vi "Get Caster Wheel Click Zones.vi"(6 "wheel frame angle (rad)":dbl, 7 "global wheel position":cluster{"x":dbl, "y":dbl}, 8 "error in (no error)":errorcluster, 9 "wheel index":i32, 11 "wheel in":refnum<class "NI_Robotics_Wheel.lvclass">) -> (0 "error out":errorcluster, 2 "click zones":T1[](array[typedef]), 3 "wheel out":refnum<class "NI_Robotics_Wheel.lvclass">)   [LabVIEW 2017, in "NI_Robotics_Configure Steering Frame.lvlib"]
uses:
  <vilib>/robotics/Dialog/Configure Steering Frame/NI_Robotics_Configure Steering Frame.lvlib
  <vilib>/robotics/Dialog/Configure Steering Frame/Click Zone.ctl
  <vilib>/robotics/Steering/Wheel/NI_Robotics_Wheel.lvclass
  <vilib>/Analysis/coordinate.llb/2D Cartesian Coordinate Rotation (Scalar).vi
  <vilib>/robotics/Steering/Wheel/Get Caster Wheel Information.vi
  <vilib>/Analysis/NI_AALPro.lvlib
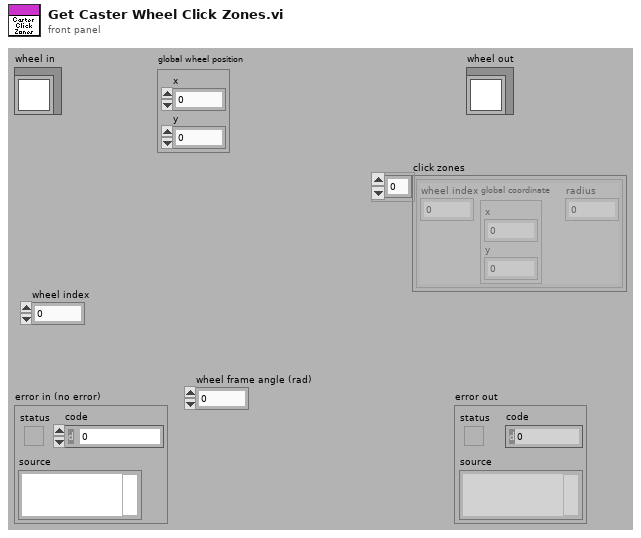
[diagram p1: front panel]
types:
  T1 = typedef "NI_Robotics_Configure Steering Frame.lvlib/Click Zone.ctl" = cluster{"wheel index":i32, "global coordinate":cluster{"x":dbl, "y":dbl}, "radius":dbl}
  T2 = typedef "NI_Robotics_Wheel.lvclass/Wheel Parameters.ctl" = cluster{"wheel radius":dbl, "gear ratio":dbl, "forward rotation direction":T3}
  T3 = typedef "NI_Robotics_Wheel.lvclass/Rotation Direction.ctl" = u16
  T4 = typedef "NI_Robotics_Caster Wheel.lvclass/Caster Wheel Parameters.ctl" = cluster{"forward offset":dbl, "caster gear ratio":dbl}
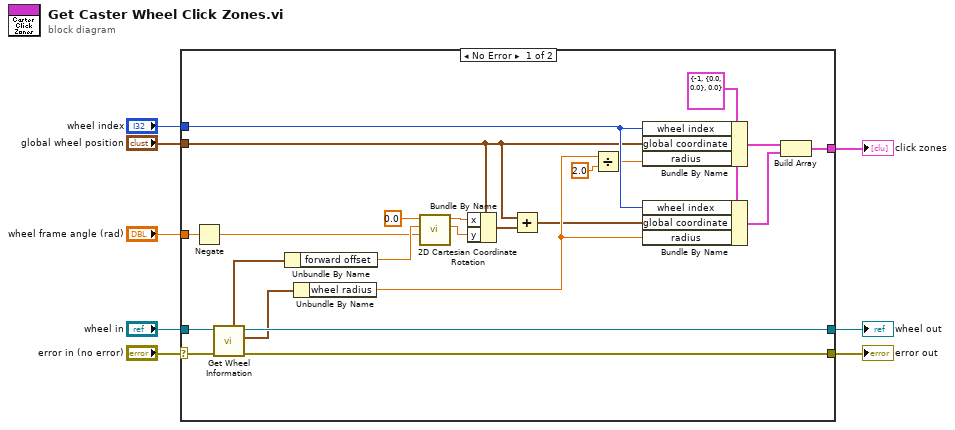
[diagram p0: block diagram]
diagram:
  n1 = case shown="No Error" "error in (no error)" {
    selector: "error in (no error)" -> [w30 w33]
    tunnel: [w29 w33] -> w2
    tunnel: "wheel in" -> [w31 w32]
    tunnel: "global wheel position" -> [w11 _]
    tunnel: [w28 w32] -> w5
    tunnel: "wheel index" -> [w26 _]
    tunnel: [w23 _] -> w7
    tunnel: "wheel frame angle (rad)" -> [w18 _]
    frame No Error {
      w9 = T1 {"wheel index"=-1, "global coordinate"={"x"=0.0, "y"=0.0}, "radius"=0.0} ("click zone")
      n2 = Negate(x=w18) -> (-x=w13:dbl)
      n3 = call-poly <vilib>:"Get Wheel Information.vi"("error in (no error)"=w30, "wheel in"=w31) -> ("error out"=w29:errorcluster, "wheel parameters"=w27:T2, "wheel out"=w28:refnum<class "NI_Robotics_Wheel.lvclass">, "caster parameters"=w19:T4)  [unwired: 3 in, 3 out]
      n4 = Unbundle By Name(w19) -> ("forward offset"=w14:dbl)
      n5 = Unbundle By Name(w27) -> ("wheel radius"=w20:dbl)
      n6 = call-poly <vilib>:"2D Cartesian Coordinate Rotation.vi"("theta"=w13, "y"=w14, "x"=0.0) -> ("y out"=w17:dbl, "x out"=w16:dbl)  [unwired: 6 in, 1 out]
      n7 = Bundle By Name(cluster=w11, "x"=w16, "y"=w17) -> (w12:cluster{"x":dbl, "y":dbl})
      n8 = Add(x=w11, y=w12) -> (x+y=w10:cluster{"x":dbl, "y":dbl})
      n9 = Divide(x=w20, y=2.0) -> (x/y=w21:dbl)
      n10 = Bundle By Name(cluster=w9, "wheel index"=w26, "global coordinate"=w11, "radius"=w21) -> (w25:T1)
      n11 = Bundle By Name(cluster=w9, "wheel index"=w26, "global coordinate"=w10, "radius"=w20) -> (w24:T1)
      n12 = Build Array(w25, w24) -> (w23:T1[])
    }
    frame Error {
    }
  }
  "error out" <- w2
  "wheel out" <- w5
  "click zones" <- w7
